vi "Configure Multi-Point.vi"(8 "error in (no error)":errorcluster, 10 "Params":variant, 11 "NI DMM in":refnum<class "NI DMM.lvclass">) -> (0 "error out":errorcluster, 3 "NI DMM out":refnum<class "NI DMM.lvclass">)   [LabVIEW 2020, in "NI DMM.lvlib" / "NI DMM.lvclass"]
uses:
  NI DMM.lvclass
  NI DMM.lvclass/NI DMM.ctl
  TypeDefs/Multi-point settings.ctl
  <instrlib>/niDMM/nidmm.llb/niDMM Sample Trigger.ctl
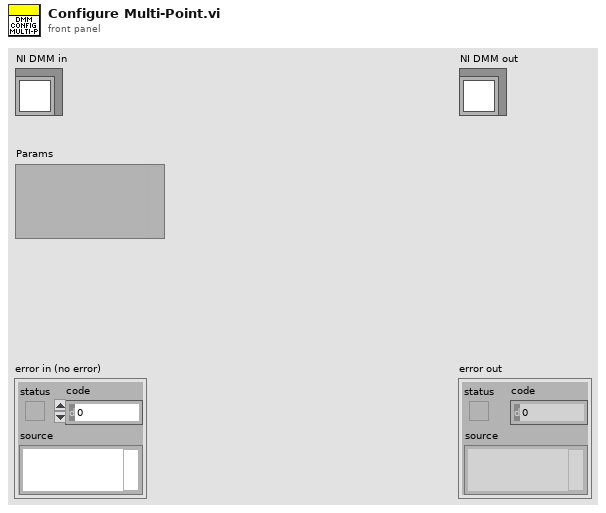
[diagram p1: front panel]
types:
  T1 = typedef "Multi-point settings.ctl" = cluster{"Sample Trigger":T2, "Trigger Count":i32, "Sample Count":i32, "Sample Interval (sec)":dbl}
  T2 = typedef "niDMM Sample Trigger.ctl" = enum16{"Immediate", "External", "TTL 0", "TTL 1", "TTL 2", "TTL 3", "TTL 4", "TTL 5", "TTL 6", "Interval", "Software", "TTL 7", "PXI Star", "LBR Trig 1", "Aux Trig 1"}
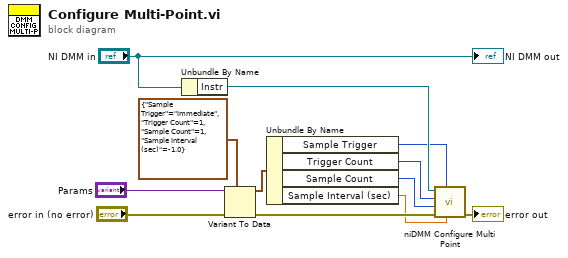
[diagram p0: block diagram]
diagram:
  n1 = Unbundle By Name("NI DMM in") -> ("Instr"=w11:refnum<k15>)
  n2 = Variant To Data(error in="error in (no error)", type=T1 {"Sample Trigger"=enum."Immediate", "Trigger Count"=1, "Sample Count"=1, "Sample Interval (sec)"=-1.0} ("Multi-point settings"), Variant="Params") -> (data=w5:T1, error out=w8:errorcluster)
  n3 = Unbundle By Name(w5) -> ("Sample Trigger"=w4:T2, "Trigger Count"=w3:i32, "Sample Count"=w2:i32, "Sample Interval (sec)"=w1:dbl)
  n4 = call <instrlib>:"niDMM Configure Multi Point.vi"("Sample Interval (sec)"=w1, "Sample Trigger"=w4, "error in (no error)"=w8, "Sample Count"=w2, "Trigger Count"=w3, "instrument handle"=w11) -> ("error out"=→"error out":errorcluster)  [unwired: 4 in, 1 out]
  "NI DMM out" <- "NI DMM in"
